vi "singleRead.vi"() -> ()   [LabVIEW 2020]
uses:
  System.Windows.Forms
panel:
  out "read channel 1":string
  out "read buffer":string
  out "Waveform Graph":i16[](graph)
  in  "error in (no error)":errorcluster
  in  "VISA resource name":refnum<visa-resource-name>
  in  "Single shot":bool
  in  "elektrotechnik2go":refnum<k24>(container)
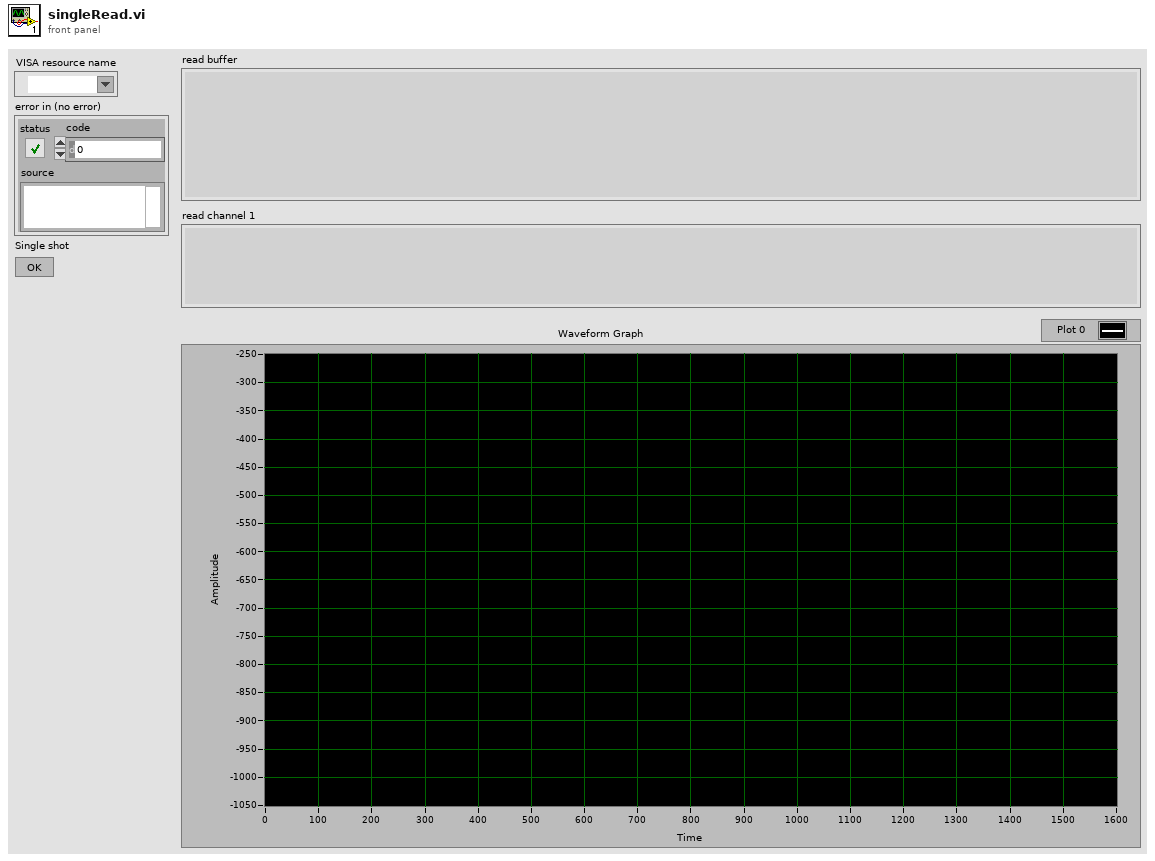
[diagram p1: front panel]
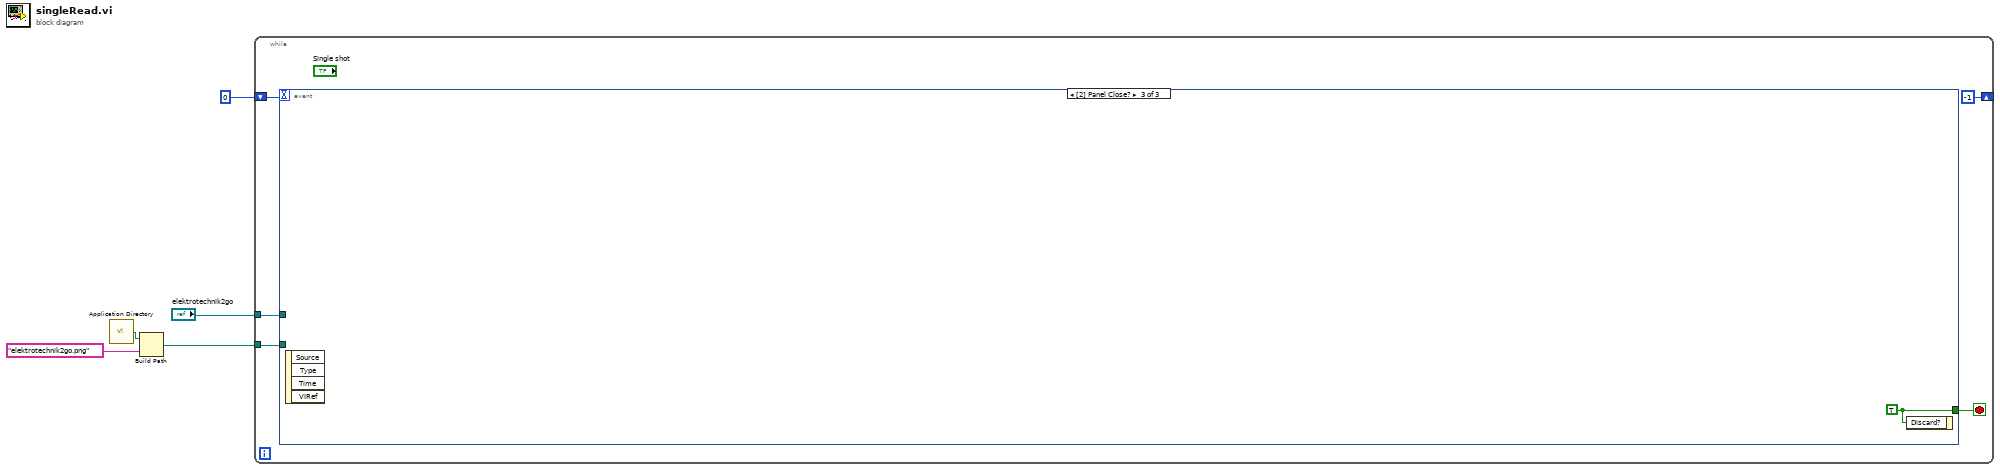
[diagram p0: block diagram]
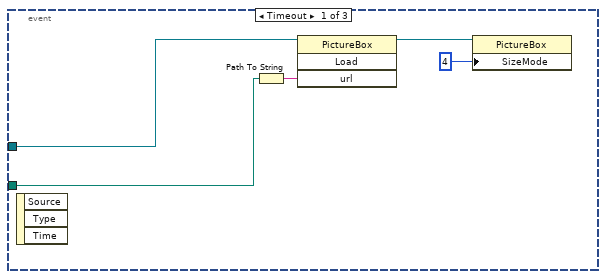
[diagram p2: hidden frame]
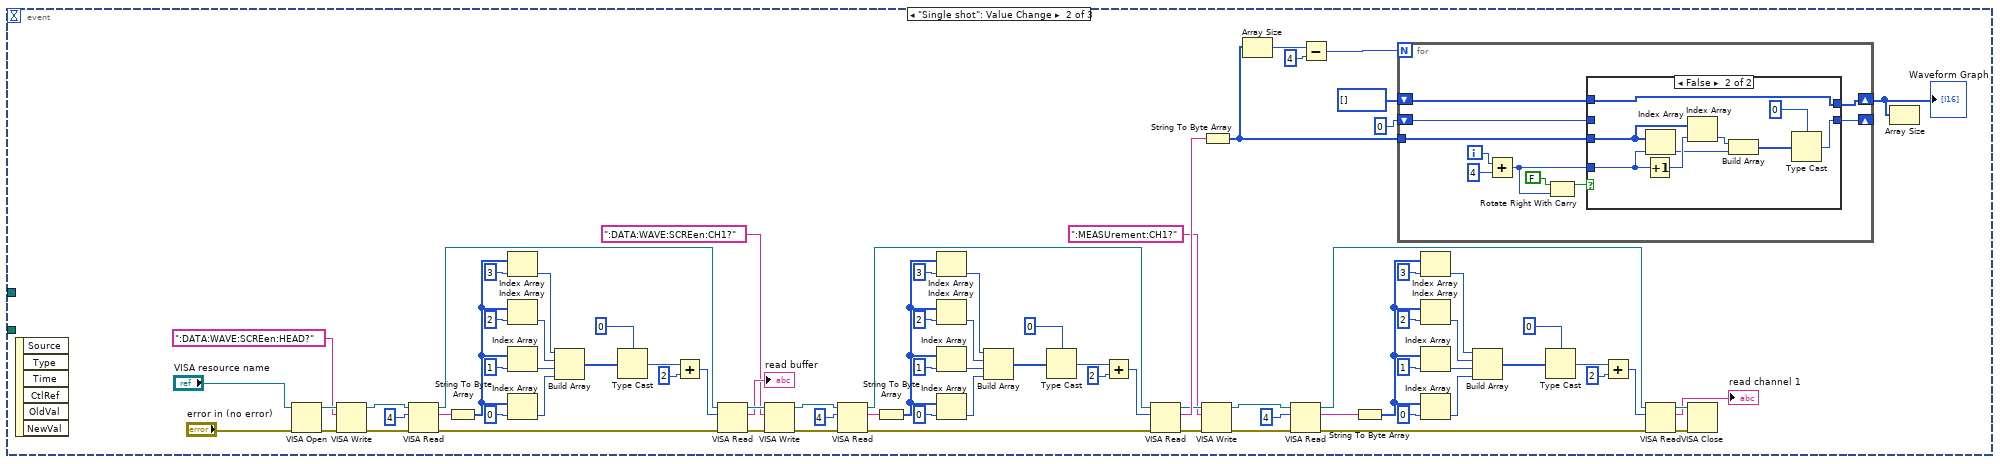
[diagram p3: hidden frame]
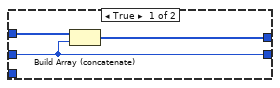
[diagram p4: hidden frame]
diagram:
  n1 = call <vilib>:"Application Directory.vi"() -> ("Application Directory"=w4:path)
  n2 = Build Path(base path=w4, name or relative path="elektrotechnik2go.png") -> (appended path=w2:path)
  n3 = while {
    tunnel: "elektrotechnik2go" -> [w9]
    tunnel: w2 -> [w8]
    shift-right: [-1] -> _
    shift-left: 0 -> [w7]
    stop <- w10 stop-if-true
    n4 = event shown="[2] Panel Close?" {
      selector: _ -> [_ _ _]
      dyn-events: _ -> [_ _ _]
      timeout: w7 -> [_ _ _]
      tunnel: [_ _ w121] -> w10
      tunnel: w9 -> [w13 _ _]
      tunnel: w8 -> [w12 _ _]
      event Timeout {
        n5 = event-data() -> ()  [unwired: 1 in, 3 out]
        n6 = Path To String(path=w12) -> (string=w15:string)
        n7 = invoke class="PictureBox" method="Load"(reference=w13, "url"=w15) -> (reference out=w14:refnum<k24>)  [unwired: 2 in, 3 out]
        n8 = property class="PictureBox"(reference=w14, "SizeMode"=4 ("Value (Signaling)")) -> ()  [unwired: 1 in, 2 out]
      }
      event "Single shot": Value Change {
        n9 = event-data() -> ()  [unwired: 1 in, 6 out]
        n10 = VISA Open(error in (no error)="error in (no error)", VISA resource name="VISA resource name") -> (VISA resource name=w90:refnum<visa-resource-name>, error out=w91:errorcluster)  [unwired: 3 in]
        n11 = VISA Write(VISA resource name=w90, write buffer=":DATA:WAVE:SCREen:HEAD?", error in (no error)=w91) -> (VISA resource name out=w41:refnum<visa-resource-name>, error out=w42:errorcluster)  [unwired: 1 out]
        n12 = VISA Read(VISA resource name=w41, byte count=u32 4, error in (no error)=w42) -> (VISA resource name out=w47:refnum<visa-resource-name>, read buffer=w55:string, error out=w46:errorcluster)  [unwired: 1 out]
        n13 = String To Byte Array(string=w55) -> (unsigned byte array=w54:u8[])
        n14 = Index Array(array=w54, index=3) -> (element=w57:u8)
        n15 = Index Array(array=w54, index=2) -> (element=w56:u8)
        n16 = Index Array(array=w54, index=1) -> (element=w51:u8)
        n17 = Index Array(array=w54, index=0) -> (element=w50:u8)
        n18 = Build Array(w57, w56, w51, w50) -> (w48:u8[])
        n19 = Type Cast(type=u32 0, x=w48) -> (*(type *) &x=w45:u32)
        n20 = Add(x=w45, y=u32 2) -> (x+y=w43:u32)
        n21 = VISA Read(VISA resource name=w47, byte count=w43, error in (no error)=w46) -> (VISA resource name out=w40:refnum<visa-resource-name>, read buffer=→"read buffer":string, error out=w38:errorcluster)  [unwired: 1 out]
        n22 = VISA Write(VISA resource name=w40, write buffer=":DATA:WAVE:SCREen:CH1?" ("Send command"), error in (no error)=w38) -> (VISA resource name out=w20:refnum<visa-resource-name>, error out=w19:errorcluster)  [unwired: 1 out]
        n23 = VISA Read(VISA resource name=w20, byte count=u32 4, error in (no error)=w19) -> (VISA resource name out=w18:refnum<visa-resource-name>, read buffer=w31:string, error out=w17:errorcluster)  [unwired: 1 out]
        n24 = String To Byte Array(string=w31) -> (unsigned byte array=w30:u8[])
        n25 = Index Array(array=w30, index=3) -> (element=w33:u8)
        n26 = Index Array(array=w30, index=2) -> (element=w32:u8)
        n27 = Index Array(array=w30, index=1) -> (element=w27:u8)
        n28 = Index Array(array=w30, index=0) -> (element=w26:u8)
        n29 = Build Array(w33, w32, w27, w26) -> (w24:u8[])
        n30 = Type Cast(type=u32 0, x=w24) -> (*(type *) &x=w23:u32)
        n31 = Add(x=w23, y=u32 2) -> (x+y=w16:u32)
        n32 = VISA Read(VISA resource name=w18, byte count=w16, error in (no error)=w17) -> (VISA resource name out=w85:refnum<visa-resource-name>, read buffer=w96:string, error out=w82:errorcluster)  [unwired: 1 out]
        n33 = VISA Write(VISA resource name=w85, write buffer=":MEASUrement:CH1?", error in (no error)=w82) -> (VISA resource name out=w84:refnum<visa-resource-name>, error out=w81:errorcluster)  [unwired: 1 out]
        n34 = String To Byte Array(string=w96) -> (unsigned byte array=w95:u8[])
        n35 = Array Size(array=w95) -> (size(s)=w88:i32)
        n36 = VISA Read(VISA resource name=w84, byte count=u32 4, error in (no error)=w81) -> (VISA resource name out=w67:refnum<visa-resource-name>, read buffer=w75:string, error out=w66:errorcluster)  [unwired: 1 out]
        n37 = Subtract(x=w88, y=4) -> (x-y=w87:i32)
        n38 = String To Byte Array(string=w75) -> (unsigned byte array=w74:u8[])
        n39 = for {
          N: w87 -> [_]
          tunnel: w95 -> [w106]
          shift-right: [w105] -> _
          shift-left: i16 0 -> [w104]
          shift-right: [w103] -> w92
          shift-left: i16[] [] -> [w102]
          i -> [w101]
          n40 = Add(x=w101, y=4) -> (x+y=w99:i32)
          n41 = Rotate Right With Carry(2:w99, 3:FALSE ("carry")) -> (1:w107:bool)  [unwired: 1 out]
          n42 = case shown="False" w107 {
            tunnel: w106 -> [_ w120]
            tunnel: w99 -> [_ w114]
            tunnel: [w109 w118] -> w105
            tunnel: w104 -> [w109 _]
            tunnel: [w111 w116] -> w103
            tunnel: w102 -> [w110 w116]
            frame True {
              n43 = Build Array (concatenate)(w110, w109) -> (w111:i16[])
            }
            frame False {
              n44 = Increment(x=w114) -> (x+1=w115:i32)
              n45 = Index Array(array=w120, index=w114) -> (element=w112:u8)
              n46 = Index Array(array=w120, index=w115) -> (element=w113:u8)
              n47 = Build Array(w113, w112) -> (w119:u8[])
              n48 = Type Cast(type=i16 0, x=w119) -> (*(type *) &x=w118:i16)
            }
          }
        }
        "Waveform Graph" <- w92
        n49 = Index Array(array=w74, index=3) -> (element=w77:u8)
        n50 = Index Array(array=w74, index=2) -> (element=w76:u8)
        n51 = Index Array(array=w74, index=1) -> (element=w71:u8)
        n52 = Index Array(array=w74, index=0) -> (element=w70:u8)
        n53 = Build Array(w77, w76, w71, w70) -> (w68:u8[])
        n54 = Type Cast(type=u32 0, x=w68) -> (*(type *) &x=w62:u32)
        n55 = Add(x=w62, y=u32 2) -> (x+y=w60:u32)
        n56 = VISA Read(VISA resource name=w67, byte count=w60, error in (no error)=w66) -> (VISA resource name out=w64:refnum<visa-resource-name>, read buffer=→"read channel 1":string, error out=w65:errorcluster)  [unwired: 1 out]
        n57 = VISA Close(VISA resource name=w64, error in (no error)=w65) -> ()  [unwired: 1 out]
        n58 = Array Size(array=w92) -> ()  [unwired: 1 out]
      }
      event Panel Close? {
        w121 = TRUE
        n59 = event-data() -> ()  [unwired: 1 in, 4 out]
        n60 = event-data("Discard?"=w121) -> ()  [unwired: 1 in, 1 out]
      }
    }
  }
